vi "Traffic-Light.vi"() -> ()   [LabVIEW 2014]
panel:
  in  "flash red":bool
  in  "stop":bool
  out "red":bool
  out "yellow":bool
  out "green":bool
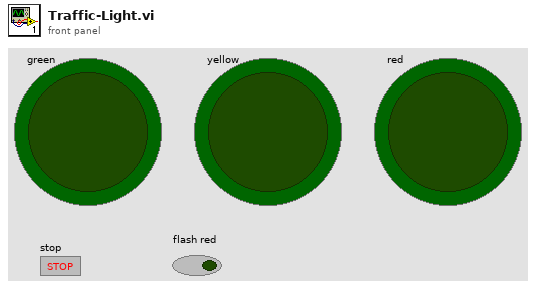
[diagram p1: front panel]
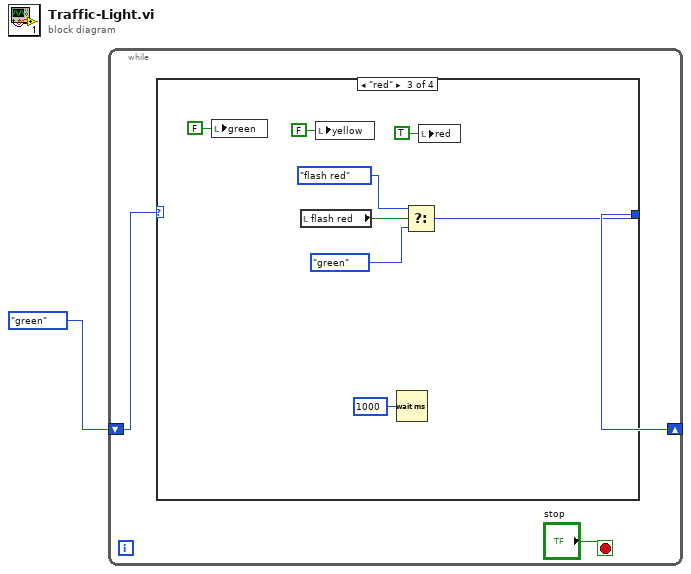
[diagram p0: block diagram]
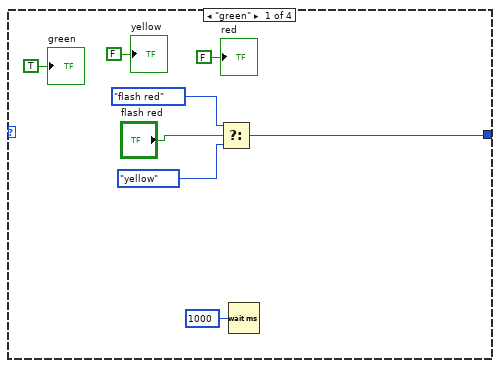
[diagram p2: hidden frame]
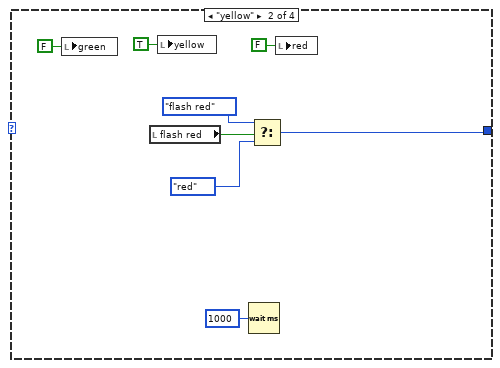
[diagram p3: hidden frame]
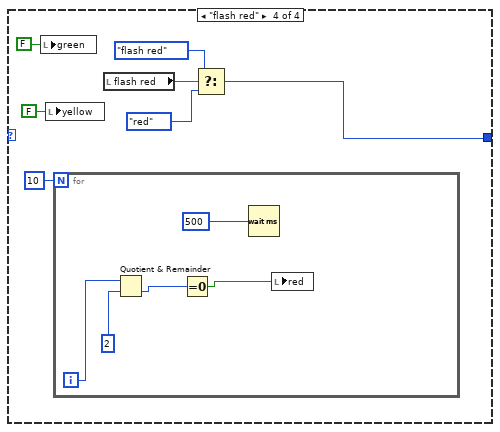
[diagram p4: hidden frame]
diagram:
  n1 = while {
    shift-right: [w3] -> _
    shift-left: enum16{"green", "yellow", "red", "flash red"}."green" -> [w2]
    stop <- "stop" stop-if-true
    n2 = case shown="\"red\"" w2 {
      tunnel: [w12 w20 w28 w35] -> w3
      frame "green" {
        n3 = Select(t=enum16{"green", "yellow", "red", "flash red"}."flash red", s="flash red", f=enum16{"green", "yellow", "red", "flash red"}."yellow") -> (s? t:f=w12:enum16{"green", "yellow", "red", "flash red"})
        n4 = Wait (ms)(milliseconds to wait=u32 1000) -> ()  [unwired: 1 out]
        "green" <- TRUE ("green")
        "yellow" <- FALSE ("yellow")
        "red" <- FALSE ("red")
      }
      frame "yellow" {
        n5 = local write "green"(FALSE ("green")) -> ()
        n6 = local read "flash red"() -> (w19:bool)
        n7 = local write "yellow"(TRUE ("yellow")) -> ()
        n8 = Wait (ms)(milliseconds to wait=u32 1000) -> ()  [unwired: 1 out]
        n9 = Select(t=enum16{"green", "yellow", "red", "flash red"}."flash red", s=w19, f=enum16{"green", "yellow", "red", "flash red"}."red") -> (s? t:f=w20:enum16{"green", "yellow", "red", "flash red"})
        n10 = local write "red"(FALSE ("red")) -> ()
      }
      frame "red" {
        n11 = local write "green"(FALSE ("green")) -> ()
        n12 = local read "flash red"() -> (w27:bool)
        n13 = local write "yellow"(FALSE ("yellow")) -> ()
        n14 = Wait (ms)(milliseconds to wait=u32 1000) -> ()  [unwired: 1 out]
        n15 = Select(t=enum16{"green", "yellow", "red", "flash red"}."flash red", s=w27, f=enum16{"green", "yellow", "red", "flash red"}."green") -> (s? t:f=w28:enum16{"green", "yellow", "red", "flash red"})
        n16 = local write "red"(TRUE ("red")) -> ()
      }
      frame "flash red" {
        n17 = local write "green"(FALSE ("green")) -> ()
        n18 = local write "yellow"(FALSE ("yellow")) -> ()
        n19 = for {
          N: 10 -> [_]
          i -> [w37]
          n20 = Quotient & Remainder(x=w37, y=2) -> (floor(x/y)=w39:i32)  [unwired: 1 out]
          n21 = Equal To 0?(x=w39) -> (x = 0?=w38:bool)
          n22 = Wait (ms)(milliseconds to wait=u32 500 ("millisecond timer value")) -> ()  [unwired: 1 out]
          n23 = local write "red"(w38) -> ()
        }
        n24 = local read "flash red"() -> (w31:bool)
        n25 = Select(t=enum16{"green", "yellow", "red", "flash red"}."flash red", s=w31, f=enum16{"green", "yellow", "red", "flash red"}."red") -> (s? t:f=w35:enum16{"green", "yellow", "red", "flash red"})
      }
    }
  }
